vi "GetTime.vi"(2 "error in":errorcluster) -> (0 "error out":errorcluster, 1 "Time":u32)   [LabVIEW 2013]
doc: "Gets the value from the millisecond timer. Meant to be synced with an error cluster for benchmarking."
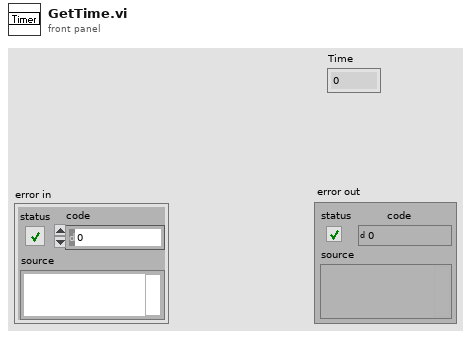
[diagram p1: front panel]
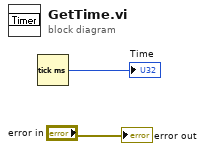
[diagram p0: block diagram]
diagram:
  n1 = Tick Count (ms)() -> (millisecond timer value=→"Time":u32)
  "error out" <- "error in"
